vi "Dictionary.Expand Array Size.vi"(8 "error in (no error)":errorcluster, 10 "Data (Dictionary)":T1[](array[typedef])) -> (0 "error out":errorcluster, 2 "Data (Dictionary)":T1[](array[typedef]))   [LabVIEW 2016, in "Conversion.lvclass"]
uses:
  Conversion.lvclass
  Data/Typedefs/Dictionary--cluster.ctl
  <vilib>/Utility/Data Type/NI_Data Type.lvlib
  Data/Data.lvclass
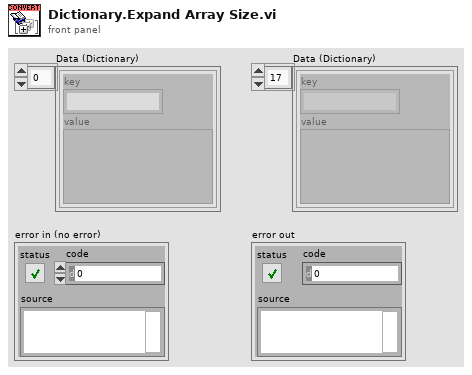
[diagram p1: front panel]
types:
  T1 = typedef "Data.lvclass/Dictionary--cluster.ctl" = cluster{"key":string, "value":variant}
  T2 = typedef "NI_Data Type.lvlib/Data Type.ctl" = enum8{"Invalid Type", "Void", "I8", "I16", "I32", "I64", "U8", "U16", "U32", "U64", "Single Float", "Double Float", "Extended Float", "Single Complex", "Double Complex", "Extended Complex", "Enum U8", "Enum U16", "Enum U32", "Enum U64", "Single Float With Unit", "Double Float With Unit", "Extended Float With Unit", "Single Complex with Unit", "Double Complex with Unit", "Extended Complex with Unit", "Boolean", "String", "Path", "Picture", "Tag", "Array", "Cluster", "Variant", "LV Variant", "Waveform", "Timestamp", "Digital Waveform", "Digital Data", "ExpressData", "Refnum", "External Data", "VI", "Poly VI", "LabVIEW Class Instance", "Fixed Point"}
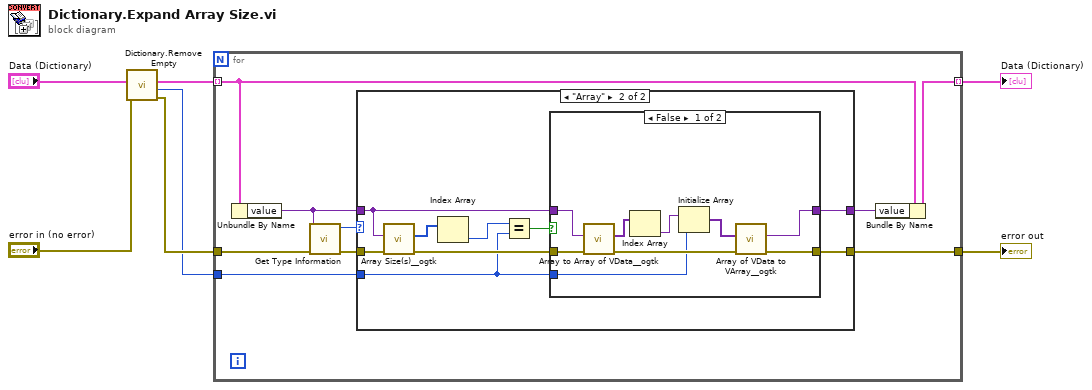
[diagram p0: block diagram]
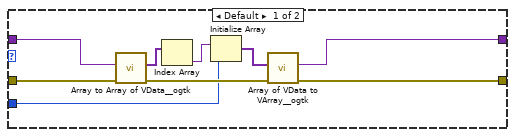
[diagram p2: hidden frame]
diagram:
  n1 = call "Dictionary.Remove Empty.vi"("error in (no error)"="error in (no error)", "Data (Dictionary)"="Data (Dictionary)") -> ("error out"=w4:errorcluster, "max Array Size"=w1:i32, "Data (Dictionary)"=w3:T1[])  [unwired: 7 in]
  n2 = for {
    tunnel: w1 -> [w13]
    tunnel: w3 -> [w9] mode=indexing
    tunnel: [w8] -> w7 mode=indexing
    tunnel: w4 -> [w16]
    tunnel: [w12] -> w6
    n3 = Unbundle By Name(w9) -> ("value"=w14:variant)
    n4 = call <vilib>:"Get Type Information.vi"("error in (no error)"=w16, "Variant"=w14) -> ("error out"=w11:errorcluster, "Type"=w15:T2)  [unwired: 5 in, 3 out]
    n5 = case shown="\"Array\"" w15 {
      tunnel: w11 -> [w21 w31]
      tunnel: w14 -> [w17 w29]
      tunnel: [w19 w33] -> w10
      tunnel: w13 -> [w18 w27]
      tunnel: [w20 w26] -> w12
      frame Default {
        n6 = call <userlib>:"Array to Array of VData__ogtk.vi"("error in (no error)"=w21, "MultiD Array"=w17) -> ("error out"=w22:errorcluster, "1D Array of Variants"=w25:variant[])  [unwired: 8 in]
        n7 = Index Array(array=w25) -> (element=w24:variant)  [unwired: 1 in]
        n8 = Initialize Array(w24, w18) -> (w23:variant[])
        n9 = call <userlib>:"Array of VData to VArray__ogtk.vi"("error in (no error)"=w22, "1D Array of VData"=w23) -> ("error out"=w20:errorcluster, "VArray"=w19:variant)  [unwired: 8 in]
      }
      frame "Array" {
        n10 = call <userlib>:"Array Size(s)__ogtk.vi"("error in (no error)"=w31, "Array"=w29) -> ("error out"=w28:errorcluster, "Size(s)"=w32:u32[])  [unwired: 7 in, 1 out]
        n11 = Index Array(array=w32) -> (element=w30:u32)  [unwired: 1 in]
        n12 = Equal?(x=w30, y=w27) -> (x = y?=w34:bool)
        n13 = case shown="False" w34 {
          tunnel: [w36 w45] -> w33
          tunnel: w29 -> [w41 w45]
          tunnel: w28 -> [w42 w44]
          tunnel: w27 -> [w37 _]
          tunnel: [w35 w44] -> w26
          frame False {
            n14 = call <userlib>:"Array to Array of VData__ogtk.vi"("error in (no error)"=w42, "MultiD Array"=w41) -> ("error out"=w38:errorcluster, "1D Array of Variants"=w43:variant[])  [unwired: 8 in]
            n15 = Index Array(array=w43) -> (element=w40:variant)  [unwired: 1 in]
            n16 = Initialize Array(w40, w37) -> (w39:variant[])
            n17 = call <userlib>:"Array of VData to VArray__ogtk.vi"("error in (no error)"=w38, "1D Array of VData"=w39) -> ("error out"=w35:errorcluster, "VArray"=w36:variant)  [unwired: 8 in]
          }
          frame True {
          }
        }
      }
    }
    n18 = Bundle By Name(cluster=w9, "value"=w10) -> (w8:T1)
  }
  "error out" <- w6
  "Data (Dictionary)" <- w7
